vi "Extendlines.vi"(11 "Start Goal Data":T1) -> (3 "Start Goal Data out":T1)   [LabVIEW 2013]
uses:
  Bug_StartGoalData.ctl
  <vilib>/Analysis/NI_AALPro.lvlib
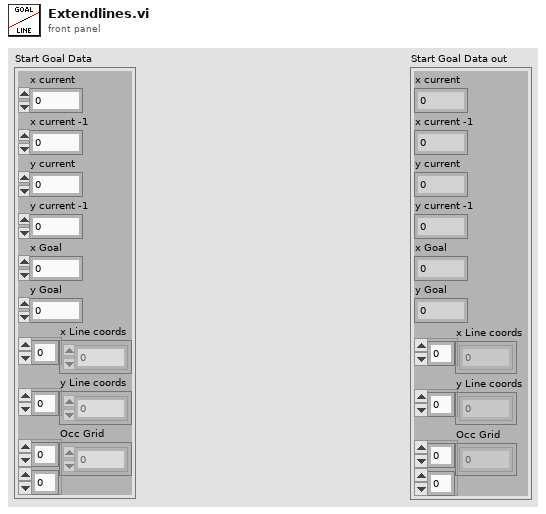
[diagram p1: front panel]
types:
  T1 = typedef "Bug_StartGoalData.ctl" = cluster{"x current":i32, "x current -1":i32, "y current":i32, "y current -1":i32, "x Goal":i32, "y Goal":i32, "x Line coords":i32[], "y Line coords":i32[], "Occ Grid":dbl[][]}
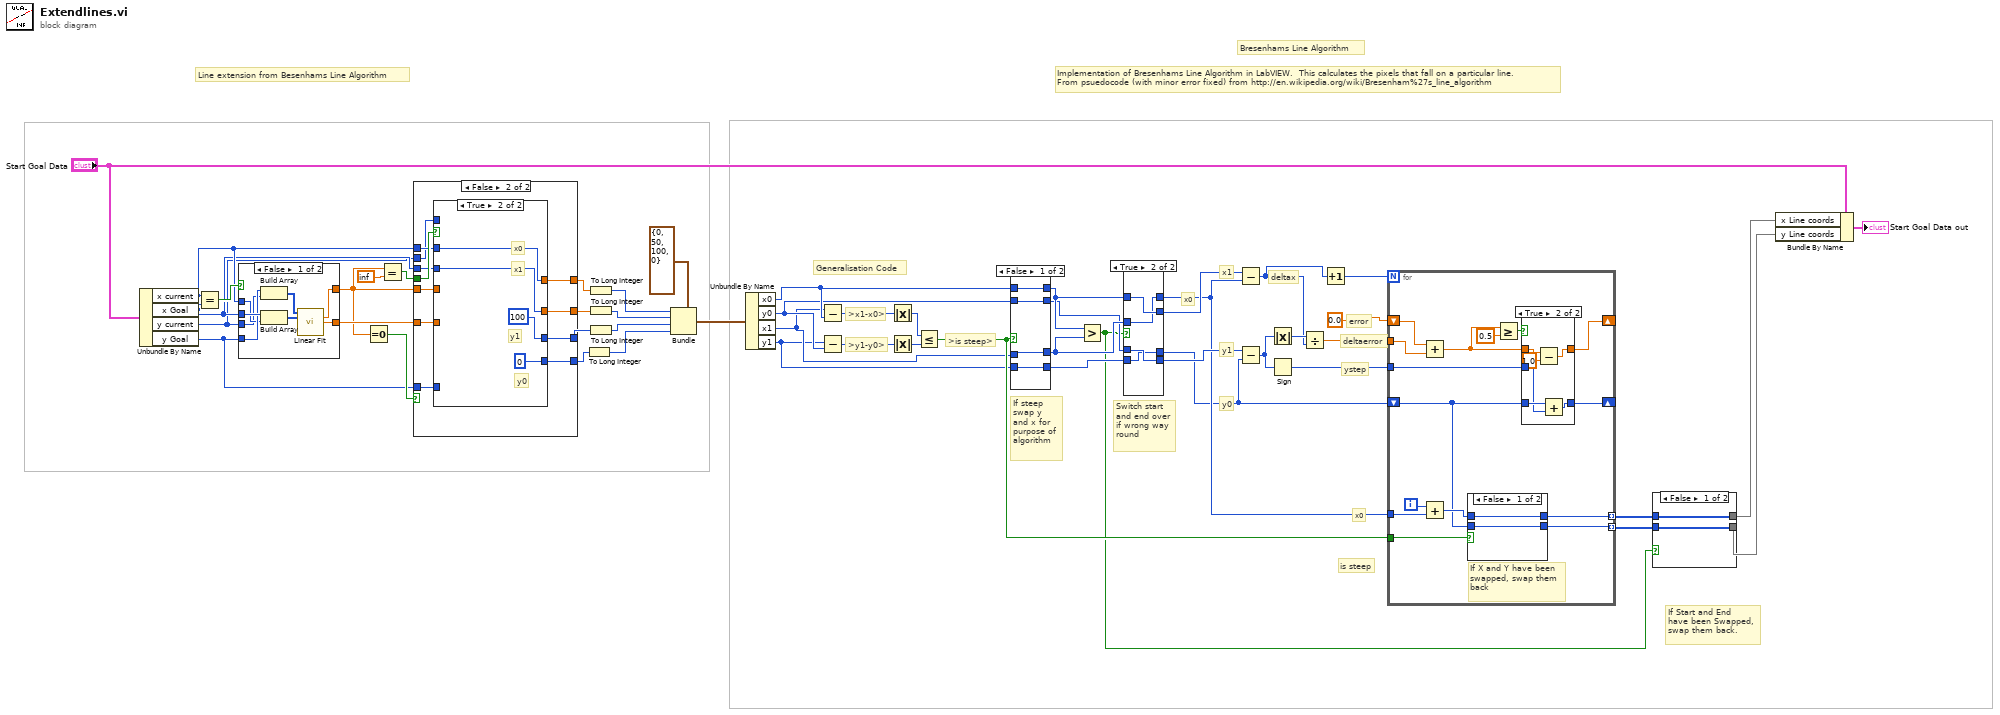
[diagram p0: block diagram]
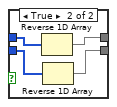
[diagram p2: hidden frame]
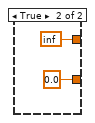
[diagram p7: hidden frame]
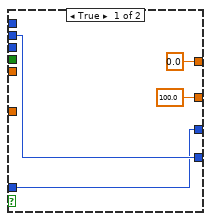
[diagram p8: hidden frame]
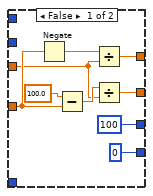
[diagram p9: hidden frame]
diagram:
  # "Line extension from Besenhams Line Algorithm"
  # "Bresenhams Line Algorithm"
  # "Implementation of Bresenhams Line Algorithm in LabVIEW.  This calculates the pixels that fall on a particular line.\nFrom psuedocode (with minor error fixed) from http://en.wikipedia.org/wiki/Bresenham%27s_line_algorithm"
  # "If Start and End\nhave been Swapped,\nswap them back."
  # "Switch start\nand end over\nif wrong way\nround"
  # "If steep\nswap y\nand x for\npurpose of\nalgorithm"
  # "is steep"
  # "x0"
  # "Generalisation Code"
  # "y0"
  # "deltaerror"
  # "error"
  # "ystep"
  # "deltax"
  # "y1"
  # "x1"
  # "x0"
  # ">is steep>"
  # ">y1-y0>"
  # ">x1-x0>"
  n1 = Unbundle By Name("Start Goal Data") -> ("x current"=w45:i32, "x Goal"=w44:i32, "y current"=w43:i32, "y Goal"=w42:i32)
  n2 = Equal?(x=w45, y=w44) -> (x = y?=w50:bool)
  n3 = case shown="False" w50 {
    tunnel: w44 -> [w59 _]
    tunnel: w42 -> [w58 _]
    tunnel: w45 -> [w57 _]
    tunnel: w43 -> [w56 _]
    tunnel: [w53 0.0 ("intercept")] -> w48
    tunnel: [w52 inf] -> w46
    frame False {
      n4 = Build Array(w58, w56) -> (w54:i32[])
      n5 = Build Array(w59, w57) -> (w55:i32[])
      n6 = call <vilib>:"Linear Fit.vi"("Y"=w54, "X"=w55) -> ("slope"=w52:dbl, "intercept"=w53:dbl)  [unwired: 9 in, 3 out]
    }
    frame True {
    }
  }
  n7 = Equal To 0?(x=w46) -> (x = 0?=w47:bool)
  n8 = Equal?(x=w46, y=inf) -> (x = y?=w51:bool)
  n9 = case shown="False" w47 {
    tunnel: w51 -> [_ w76]
    tunnel: [w62 w75] -> w39
    tunnel: [w63 w74] -> w38
    tunnel: w43 -> [w63 w69]
    tunnel: w42 -> [w62 w68]
    tunnel: w45 -> [_ w72]
    tunnel: w44 -> [_ w70]
    tunnel: [0.0 w73] -> w41
    tunnel: [100.0 w71] -> w40
    tunnel: w46 -> [_ w67]
    tunnel: w48 -> [_ w66]
    frame True {
    }
    frame False {
      n10 = case shown="True" w76 {
        tunnel: [100 100] -> w75
        tunnel: [0 0] -> w74
        tunnel: [w77 w87] -> w73
        tunnel: w72 -> [_ w87]
        tunnel: [w80 w86] -> w71
        tunnel: w70 -> [_ w86]
        tunnel: w69 -> [_ _]
        tunnel: w68 -> [_ _]
        tunnel: w67 -> [w78 _]
        tunnel: w66 -> [w83 _]
        frame False {
          n11 = Negate(x=w83) -> (-x=w79:dbl)
          n12 = Subtract(x=100.0, y=w83) -> (x-y=w81:dbl)
          n13 = Divide(x=w79, y=w78) -> (x/y=w77:dbl)
          n14 = Divide(x=w81, y=w78) -> (x/y=w80:dbl)
        }
        frame True {
          # "y1"
          # "y0"
          # "x1"
          # "x0"
        }
      }
    }
  }
  n15 = To Long Integer(number=w38) -> (32bit integer=w37:i32)
  n16 = To Long Integer(number=w41) -> (32bit integer=w34:i32)
  n17 = To Long Integer(number=w40) -> (32bit integer=w35:i32)
  n18 = To Long Integer(number=w39) -> (32bit integer=w36:i32)
  n19 = Bundle(cluster=cluster{"x0":i32, "x1":i32, "y1":i32, "y0":i32} {"x0"=0, "x1"=50, "y1"=100, "y0"=0} ("startgoal_calcout 2"), "x0"=w34, "x1"=w35, "y1"=w36, "y0"=w37) -> (w5:cluster{"x0":i32, "x1":i32, "y1":i32, "y0":i32})
  n20 = Unbundle By Name(w5) -> ("x0"=w10:i32, "y0"=w9:i32, "x1"=w8:i32, "y1"=w7:i32)
  n21 = Subtract(x=w8, y=w10) -> (x-y=w33:i32)
  n22 = Subtract(x=w7, y=w9) -> (x-y=w32:i32)
  n23 = Absolute Value(x=w33) -> (abs(x)=w30:i32)
  n24 = Absolute Value(x=w32) -> (abs(x)=w31:i32)
  n25 = Less Or Equal?(x=w30, y=w31) -> (x <= y?=w16:bool)
  n26 = case shown="False" w16 {
    tunnel: w10 -> [w93 w97]
    tunnel: w8 -> [w92 w96]
    tunnel: w9 -> [w91 w95]
    tunnel: w7 -> [w90 w94]
    tunnel: [w91 w97] -> w27
    tunnel: [w90 w96] -> w26
    tunnel: [w93 w95] -> w29
    tunnel: [w92 w94] -> w28
    frame False {
    }
    frame True {
    }
  }
  n27 = Greater?(x=w29, y=w28) -> (0:w13:bool)
  n28 = case shown="True" w13 {
    tunnel: w29 -> [w101 w105]
    tunnel: w28 -> [w100 w104]
    tunnel: w27 -> [w99 w103]
    tunnel: w26 -> [w98 w102]
    tunnel: [w101 w104] -> w21
    tunnel: [w100 w105] -> w25
    tunnel: [w99 w102] -> w18
    tunnel: [w98 w103] -> w24
    frame False {
    }
    frame True {
    }
  }
  n29 = Subtract(x=w25, y=w21) -> (x-y=w15:i32)
  n30 = Subtract(x=w24, y=w18) -> (x-y=w22:i32)
  n31 = Absolute Value(x=w22) -> (abs(x)=w23:i32)
  n32 = Sign(1:w22) -> (0:w17:i32)
  n33 = Divide(x=w23, y=w15) -> (x/y=w19:dbl)
  n34 = Increment(x=w15) -> (x+1=w14:i32)
  n35 = for {
    N: w14 -> [_]
    tunnel: w21 -> [w119]
    shift-right: [w109] -> _
    shift-left: 0.0 -> [w110]
    tunnel: w19 -> [w118]
    tunnel: w17 -> [w112]
    tunnel: w16 -> [w117]
    shift-right: [w111] -> _
    shift-left: w18 -> [w113]
    tunnel: [w107] -> w12 mode=indexing
    tunnel: [w106] -> w11 mode=indexing
    i -> [w120]
    # "If X and Y have been\nswapped, swap them\nback"
    n36 = Add(x=w110, y=w118) -> (x+y=w108:dbl)
    n37 = Add(x=w120, y=w119) -> (x+y=w116:i32)
    n38 = case shown="False" w117 {
      tunnel: w113 -> [w129 w132]
      tunnel: [w130 w132] -> w107
      tunnel: w116 -> [w130 w131]
      tunnel: [w129 w131] -> w106
      frame False {
      }
      frame True {
      }
    }
    n39 = Greater Or Equal?(x=w108, y=0.5) -> (x >= y?=w115:bool)
    n40 = case shown="True" w115 {
      tunnel: w113 -> [w121 w128]
      tunnel: w112 -> [_ w125]
      tunnel: [w121 w127] -> w111
      tunnel: w108 -> [w122 w126]
      tunnel: [w122 w124] -> w109
      frame False {
      }
      frame True {
        n41 = Subtract(x=w126, y=1.0) -> (x-y=w124:dbl)
        n42 = Add(x=w128, y=w125) -> (x+y=w127:i32)
      }
    }
  }
  n43 = case shown="False" w13 {
    tunnel: [w134 w138] -> w4
    tunnel: w12 -> [w134 w137]
    tunnel: w11 -> [w133 w136]
    tunnel: [w133 w135] -> w3
    frame False {
    }
    frame True {
      n44 = Reverse 1D Array(array=w137) -> (reversed array=w138:i32[])
      n45 = Reverse 1D Array(array=w136) -> (reversed array=w135:i32[])
    }
  }
  n46 = Bundle By Name(cluster="Start Goal Data", "x Line coords"=w4, "y Line coords"=w3) -> (→"Start Goal Data out":T1)
